vi "Postgres Example.vi"() -> ()   [LabVIEW 2020, in "ORM_Examples.lvlib"]
uses:
  ORM_Examples.lvlib
  <vilib>/Viviota/shared/ORM_ADONet.lvlibp/ADOMapper/ADOMapper.lvclass
  C:/Program Files/National Instruments/LabVIEW 2020/vi.lib/Viviota/shared/ORM.lvlibp/ORM/SqlMapper/SqlMapper.lvclass
  DbConnections/PostgresqlConnection/Postgresql Connect.vi
  ORM_API/ORM_API.lvlib
  7567ee1f-f747-46f7-b4dd-0c9fb0e63776.vi
  AlbumMap/AlbumMap.lvclass
  Album/Album.lvclass
  df564c15-4522-450c-b99f-f01b994daeb7.vi
  DbConnections/PostgresqlConnection/DBC.lvclass
  C:/Program Files/National Instruments/LabVIEW 2020/vi.lib/Viviota/shared/ORM_ADONet.lvlibp/ADOMapper/ADOMapper.lvclass
panel:
  out "error out":errorcluster
  out "id":variant
  out "Title 2":string
  out "Primary Key":i64
  in  "Title":string
  out "Value":variant
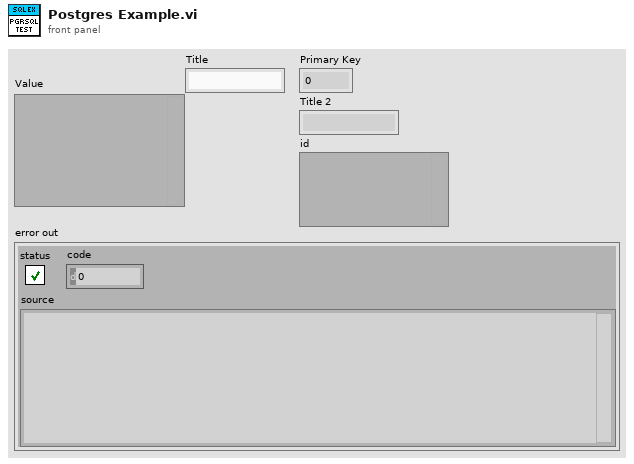
[diagram p1: front panel]
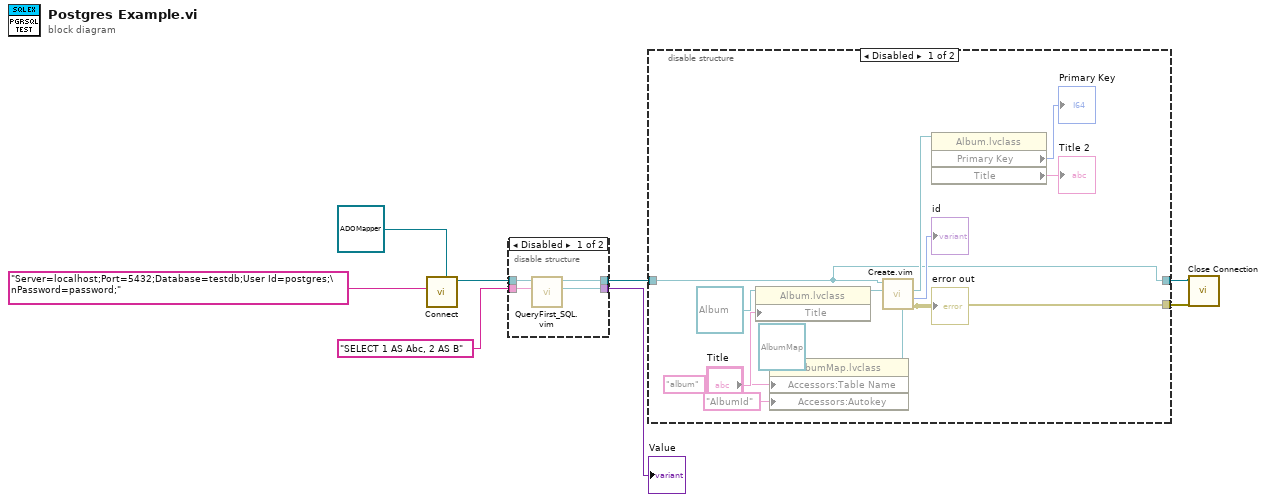
[diagram p0: block diagram]
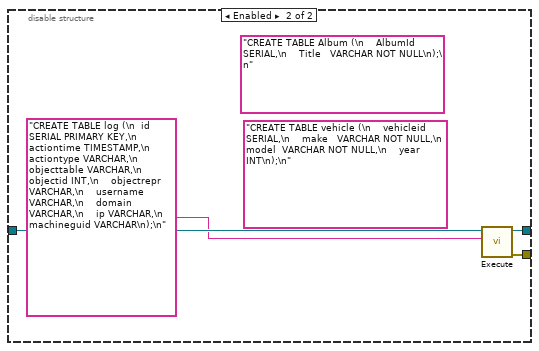
[diagram p3: hidden frame]
diagram:
  n1 = call-poly "Connect.vi"("SqlMapper Type"=refnum<class "ADOMapper.lvclass"> refnum ("ADONet.lvlib:ADOMapper.lvclass"), "Connection String"="Server=localhost;Port=5432;Database=testdb;User Id=postgres;\nPassword=password;") -> ("SqlMapper out"=w7:refnum<class "ADOMapper.lvclass">)  [unwired: 8 in, 1 out]
  n2 = disable-structure shown="Disabled" {
    disable-tunnel: w7 -> [w12 w13]
    disable-tunnel: "SELECT 1 AS Abc, 2 AS B" ("sql") -> [w11 _]
    disable-tunnel: [w10 _] -> w5
    disable-tunnel: [w9 w13] -> w4
    frame Disabled {
      n3 = call "QueryFirst_SQL.vim"("sql"=w11, "SqlMapper in"=w12) -> ("Value"=w10:refnum<class>, "SqlMapper out"=w9:refnum<class "ADOMapper.lvclass">)  [unwired: 7 in, 1 out]
    }
    frame Enabled {
    }
  }
  "Value" <- w5
  n4 = disable-structure shown="Disabled" {
    disable-tunnel: w4 -> [w14 w30]
    disable-tunnel: [w14 w28] -> w2
    disable-tunnel: [w15 w27] -> w1
    frame Disabled {
      n5 = property class="Album.lvclass"(reference=refnum<class "Album.lvclass"> refnum ("Album.lvclass"), "Title"="Title") -> (reference out=w23:refnum<class "Album.lvclass">)  [unwired: 1 in, 1 out]
      n6 = property class="AlbumMap.lvclass"(reference=refnum<class "AlbumMap.lvclass"> refnum ("AlbumMap.lvclass"), "Accessors:Table Name"="album" ("Log Table Name"), "Accessors:Autokey"="AlbumId" ("Autokey")) -> (reference out=w18:refnum<class "AlbumMap.lvclass">)  [unwired: 1 in, 1 out]
      n7 = call "Create.vim"("TypeMap in"=w18, "object in"=w23, "SqlMapper in"=w14) -> ("error out"=w15:errorcluster, "id"=→"id":i32, "object out"=w22:refnum<class "Album.lvclass">)  [unwired: 5 in, 1 out]
      "error out" <- w15
      n8 = property class="Album.lvclass"(reference=w22) -> ("Primary Key"=→"Primary Key":i64, "Title"=→"Title 2":string)  [unwired: 1 in, 2 out]
    }
    frame Enabled {
      (unwired) "CREATE TABLE vehicle (\n    vehicleid SERIAL,\n    make   VARCHAR NOT NULL,\n    model  VARCHAR NOT NULL,\n    year   INT\n);\n" ("sql")
      (unwired) "CREATE TABLE Album (\n    AlbumId SERIAL,\n    Title   VARCHAR NOT NULL\n);\n" ("sql")
      n9 = call-dynamic "Execute.vi"("sql"="CREATE TABLE log (\n  id SERIAL PRIMARY KEY,\n    actiontime TIMESTAMP,\n    actiontype VARCHAR,\n    objecttable VARCHAR,\n    objectid INT,\n    objectrepr VARCHAR,\n    username VARCHAR,\n    domain VARCHAR,\n    ip VARCHAR,\n    machineguid VARCHAR\n);\n", "ADOMapper in"=w30) -> ("error out"=w27:errorcluster, "ADOMapper out"=w28:refnum<class "ADOMapper.lvclass">)  [unwired: 7 in, 1 out]
    }
  }
  n10 = call "Close Connection.vi"("Error In"=w1, "SqlMapper"=w2) -> ()  [unwired: 9 in, 1 out]
